vi "Return_VXM_Home_win7.vi"(1 "error in (no error)":errorcluster) -> (0 "error out":errorcluster)   [LabVIEW 2017]
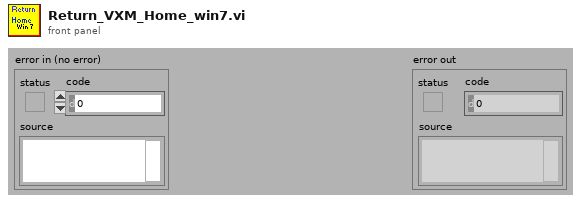
[diagram p1: front panel]
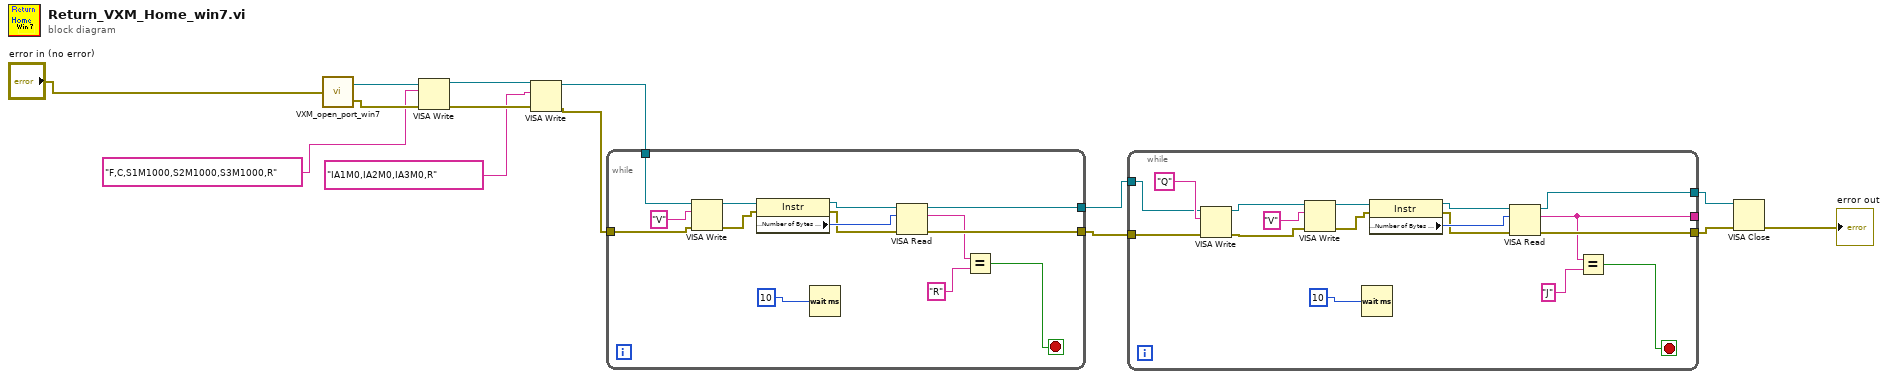
[diagram p0: block diagram]
diagram:
  n1 = call "VXM_open_port_win7.vi"("error in (no error)"="error in (no error)") -> ("VISA resource name out"=w14:refnum<visa-resource-name>, "error out"=w13:errorcluster)
  n2 = VISA Write(VISA resource name=w14, write buffer="F,C,S1M1000,S2M1000,S3M1000,R", error in (no error)=w13) -> (VISA resource name out=w10:refnum<visa-resource-name>, error out=w9:errorcluster)  [unwired: 1 out]
  n3 = VISA Write(VISA resource name=w10, write buffer="IA1M0,IA2M0,IA3M0,R", error in (no error)=w9) -> (VISA resource name out=w5:refnum<visa-resource-name>, error out=w6:errorcluster)  [unwired: 1 out]
  n4 = while {
    tunnel: w6 -> [w25]
    tunnel: w5 -> [w24]
    tunnel: [w20] -> w3
    tunnel: [w15] -> w4
    stop <- w17 stop-if-true
    n5 = VISA Write(VISA resource name=w24, write buffer="V", error in (no error)=w25) -> (VISA resource name out=w27:refnum<visa-resource-name>, error out=w26:errorcluster)  [unwired: 1 out]
    n6 = property class="Instr"(reference=w27, error in=w26) -> (reference out=w22:refnum<visa-resource-name>, error out=w21:errorcluster, "Serial Settings:Number of Bytes at Serial Port"=w23:u32)
    n7 = Wait (ms)(milliseconds to wait=10) -> ()  [unwired: 1 out]
    n8 = VISA Read(VISA resource name=w22, byte count=w23, error in (no error)=w21) -> (VISA resource name out=w15:refnum<visa-resource-name>, read buffer=w18:string, error out=w20:errorcluster)  [unwired: 1 out]
    n9 = Equal?(x=w18, y="R") -> (x = y?=w17:bool)
  }
  n10 = while {
    tunnel: [w36] -> _
    tunnel: [w39] -> w2
    tunnel: [w38] -> w1
    tunnel: w4 -> [w31]
    tunnel: w3 -> [w32]
    stop <- w35 stop-if-true
    n11 = VISA Write(VISA resource name=w31, write buffer="Q", error in (no error)=w32) -> (VISA resource name out=w30:refnum<visa-resource-name>, error out=w29:errorcluster)  [unwired: 1 out]
    n12 = VISA Write(VISA resource name=w30, write buffer="V", error in (no error)=w29) -> (VISA resource name out=w44:refnum<visa-resource-name>, error out=w43:errorcluster)  [unwired: 1 out]
    n13 = Wait (ms)(milliseconds to wait=10) -> ()  [unwired: 1 out]
    n14 = property class="Instr"(reference=w44, error in=w43) -> (reference out=w41:refnum<visa-resource-name>, error out=w40:errorcluster, "Serial Settings:Number of Bytes at Serial Port"=w42:u32)
    n15 = VISA Read(VISA resource name=w41, byte count=w42, error in (no error)=w40) -> (VISA resource name out=w39:refnum<visa-resource-name>, read buffer=w36:string, error out=w38:errorcluster)  [unwired: 1 out]
    n16 = Equal?(x=w36, y="J") -> (x = y?=w35:bool)
  }
  n17 = VISA Close(VISA resource name=w2, error in (no error)=w1) -> (error out=→"error out":errorcluster)
